vi "Example - SLL Table.vi"() -> ()   [LabVIEW 2019, in "SLL Table.lvclass"]
doc: "Example for SLL Table which deals with data manipulation."
uses:
  SLL Table.lvclass
  _Typedefs/ColumnConditionCluster.ctl
  _SubVIs/Get Table Data.vi
  _SubVIs/Get Row Data.vi
panel:
  out "Row Map":map{string, string}(c390)
  in  "Row Index":i32=1
  out "Header Order[]":string[](array[string])
  out "Count Rows[][]":string[][](array[string])
  out "2D Data[][]":string[][](array[string])
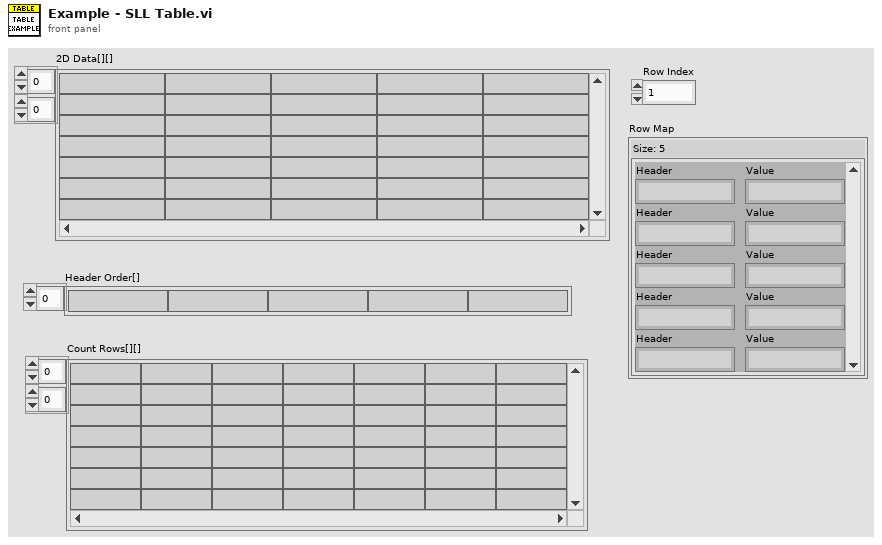
[diagram p1: front panel]
types:
  T1 = typedef "SLL Table.lvclass/ColumnConditionCluster.ctl" = cluster{"Header":string, "Value[]":string[]}
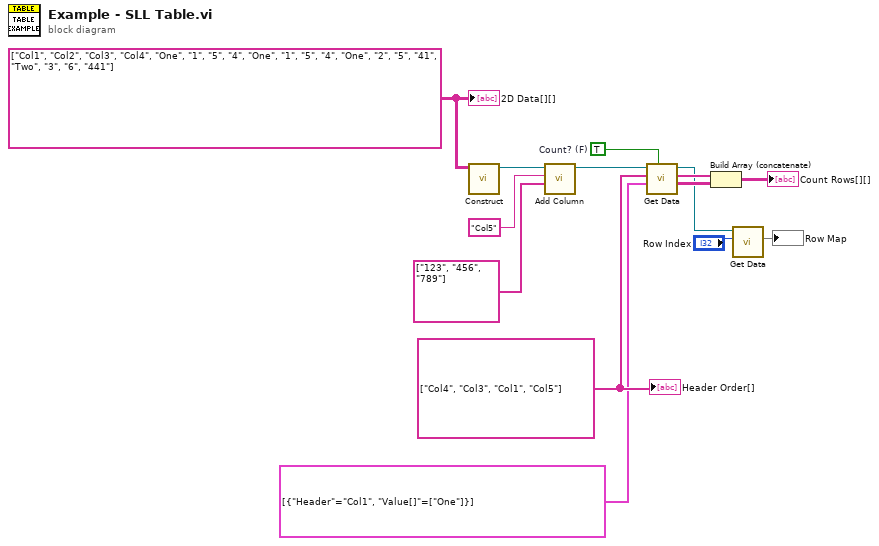
[diagram p0: block diagram]
diagram:
  w11 = TRUE  # Count? (F)
  w13 = string[] ["Col4", "Col3", "Col1", "Col5"] ("Header Order[] (Optional)")
  w5 = string[][] [["Col1", "Col2", "Col3", "Col4"], ["One", "1", "5", "4"], ["One", "1", "5", "4"], ["One", "2", "5", "41"], ["Two", "3", "6", "441"]] ("2D String with Headers")
  n1 = call "Construct.vi"("2D String with Headers"=w5) -> ("Table"=w9:refnum<class "SLL Table.lvclass">)  [unwired: 9 in, 1 out]
  n2 = call "Add Column.vi"("Data[]"=string[] ["123", "456", "789"], "Header"="Col5", "SLL Table in"=w9) -> ("SLL Table out"=w8:refnum<class "SLL Table.lvclass">)  [unwired: 7 in, 1 out]
  n3 = call-poly "Get Data.vi"("Count? (F)"=w11, "Column Conditions[] (Optional)"=T1[] [{"Header"="Col1", "Value[]"=["One"]}], "Header Order[] (Optional)"=w13, "SLL Table in"=w8) -> ("2D Data Out[][]"=w6:string[][], "Headers Out[]"=w7:string[], "SLL Table out"=w3:refnum<class "SLL Table.lvclass">)  [unwired: 4 in, 1 out]
  n4 = Build Array (concatenate)(w7, w6) -> (→"Count Rows[][]":string[][])
  n5 = call-poly "Get Data.vi"("Row Index"="Row Index", "SLL Table in"=w3) -> ("Row Map"=→"Row Map":map{string, string})  [unwired: 7 in, 2 out]
  "2D Data[][]" <- w5
  "Header Order[]" <- w13
